vi "Pos_window bounds to size.vi"(3 "Bounds":T1) -> (1 "Size":cluster{"Width":i16, "Height":i16})   [LabVIEW 2020]
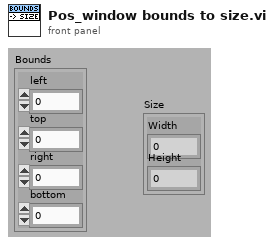
[diagram p1: front panel]
types:
  T1 = cluster{"left":i16, "top":i16, "right":i16, "bottom":i16}
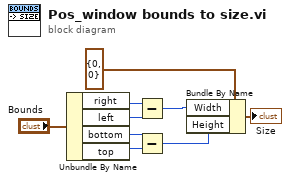
[diagram p0: block diagram]
diagram:
  n1 = Unbundle By Name("Bounds") -> ("right"=w9:i16, "left"=w8:i16, "bottom"=w7:i16, "top"=w6:i16)
  n2 = Subtract(x=w9, y=w8) -> (x-y=w5:i16)
  n3 = Subtract(x=w7, y=w6) -> (x-y=w4:i16)
  n4 = Bundle By Name(cluster=cluster{"Width":i16, "Height":i16} {"Width"=0, "Height"=0} ("Size"), "Width"=w5, "Height"=w4) -> (→"Size":cluster{"Width":i16, "Height":i16})
